vi "Angle fine search.vi"(6 "Process merged pattern":dbl[](array[numeric]), 7 "Template merged pattern":dbl[](array[numeric]), 10 "Angle step size\n(in degrees)":dbl, 11 "Angle range\n(in degrees)":dbl) -> (2 "Selected FOM":dbl, 3 "Angle correction":dbl)   [LabVIEW 2019]
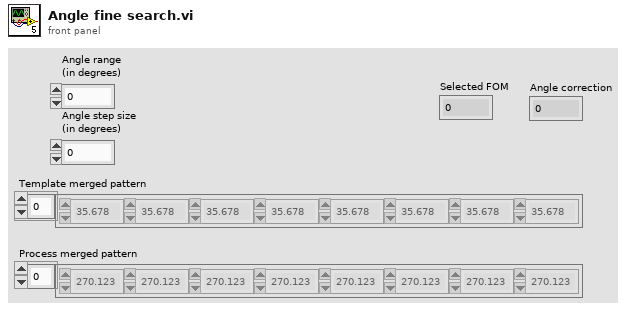
[diagram p1: front panel]
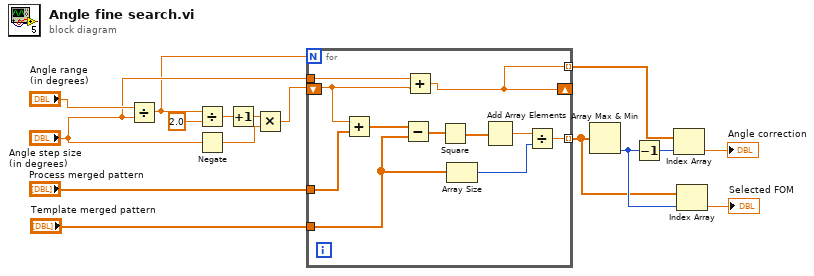
[diagram p0: block diagram]
diagram:
  n1 = Divide(x="Angle range\n(in degrees)", y="Angle step size\n(in degrees)") -> (x/y=w9:dbl)
  n2 = Divide(x=w9, y=2.0) -> (x/y=w6:dbl)
  n3 = Negate(x="Angle step size\n(in degrees)") -> (-x=w14:dbl)
  n4 = Increment(x=w6) -> (x+1=w5:dbl)
  n5 = Multiply(x=w5, y=w14) -> (x*y=w13:dbl)
  n6 = for {
    N: w9 -> [_]
    tunnel: "Process merged pattern" -> [w27]
    tunnel: "Template merged pattern" -> [w22]
    tunnel: [w20] -> w2 mode=indexing
    tunnel: "Angle step size\n(in degrees)" -> [w18]
    shift-right: [w17] -> _
    shift-left: w13 -> [w19]
    tunnel: [w17] -> w8 mode=indexing
    n7 = Add(x=w19, y=w27) -> (x+y=w26:dbl[])
    n8 = Subtract(x=w26, y=w22) -> (x-y=w25:dbl[])
    n9 = Add(x=w18, y=w19) -> (x+y=w17:dbl)
    n10 = Square(x=w25) -> (x^2=w24:dbl[])
    n11 = Array Size(array=w22) -> (size(s)=w21:i32)
    n12 = Add Array Elements(numeric array=w24) -> (sum=w23:dbl)
    n13 = Divide(x=w23, y=w21) -> (x/y=w20:dbl)
  }
  n14 = Array Max & Min(array=w2) -> (min index (indices)=w3:i32)  [unwired: 3 out]
  n15 = Decrement(x=w3) -> (x-1=w4:i32)
  n16 = Index Array(array=w8, index=w4) -> (element=→"Angle correction":dbl)
  n17 = Index Array(array=w2, index=w3) -> (element=→"Selected FOM":dbl)
